vi "Unicode String Normalization Example.vi"() -> ()   [LabVIEW 2020]
doc: "This example demonstrates Unicode string normalization and compares the result of each of the normalization forms."
uses:
  Types/UTF-8 String/UTF-8 String.lvclass/UTF-8 String.ctl
  String/Controls/Normalized Form.ctl
  Dialog & User Interface/Polymorphic VIs/Write Control Text/Write String Value (UTF-8 String).vi
  Dialog & User Interface/Polymorphic VIs/Write Control Text/Write Ring Strings (UTF-8 String).vi
  87eab71b-edd1-4ab4-a82b-cc44d71eae5a.vi
  fbd87bf1-22c2-4bfe-9a71-b40242120771.vi
  c0d17205-3000-44ff-8427-9931fc65464d.vi
  1d2ce790-e22e-409d-a6eb-9d15f9dc24c3.vi
  2fb06fa7-1877-45b3-88e1-542f5745c524.vi
  90507d11-c02e-49ea-b453-6dce07ba0123.vi
  61f88bc1-4490-4656-bc91-370f28d961b2.vi
  2387616d-ad84-49dc-88c3-6113dd534e76.vi
  364c4283-3d14-4df8-9c3b-6263318f94ac.vi
  Unicode/Encode String.vi
  Dialog & User Interface/Polymorphic VIs/Write Control Text/Write String Value (UTF-8 String).vi/5206cb6b-04fb-41f5-a37e-29c14f142303.vi
  Private/Library/gu_codepoint_array_to_string.vi
  Types/UTF-8 String/Write Encoded UTF-8 String.vi
  Dialog & User Interface/Polymorphic VIs/Write Control Text/Write Ring Strings (UTF-8 String).vi/5206cb6b-04fb-41f5-a37e-29c14f142303.vi
  Private/Library/gu_normalize_string.vi
  Private/Conversion/String as Encoded String.vi
  Private/Conversion/Polymorphic VIs/String as Encoded String (UTF-8 String).vi
  Private/Library/gu_string_to_codepoint_array.vi
  Private/Conversion/Text to UTF-8.vi
  Private/Conversion/Polymorphic VIs/Text to UTF-8 (LabVIEW String).vi
  Private/Conversion/Encoded UTF-8 String to Encoded UTF-16LE String.vi
  Unicode/SubVIs/UTF-16 Byte Swap.vi
  Private/Conversion/UTF-8 to Text.vi
  Private/Conversion/Polymorphic VIs/UTF-8 to Text (LabVIEW String).vi
  Private/Conversion/Encoded UTF-16LE String to Encoded UTF-8 String.vi
  Unicode/Prepend BOM.vi
  Private/Conversion/Text as Encoded String.vi
  Private/Conversion/Polymorphic VIs/Text as Encoded String (UTF-8 String).vi
  Private/Library/Result To Error.vi
  Private/Memory/Copy String.vi
  Types/UTF-8 String/Read Encoded UTF-8 String.vi
  Private/Library/gu_string_to_codepoint_array.vi/5c793459-c97f-49eb-b871-f007f412847a.vi
  Unicode/SubVIs/Byte Order Marks.vi
  Unicode/Detect BOM.vi
  Private/Memory/Copy String.vi/4d47babd-4a2d-4eb7-b91b-7e707d692665.vi
  Private/Library/gu_free.vi
  Private/Library/gu_string_to_codepoint_array.vi/5c793459-c97f-49eb-b871-f007f412847a.vi/bf7dd0c3-7326-468c-a5c4-9eb034008d84.vi
  Unicode/Detect String Encoding.vi
  <vilib>/Utility/error.llb/Error Cluster From Error Code.vi
  Private/User Interface/Write Ring Control.vi
  Private/User Interface/Write String.vi
  Types/UTF-8 String/UTF-8 String.lvclass
  G-Unicode.lvlib
panel:
  out "Source":cluster{"Source":i32, "Source":string}[](array[cluster]) {"Source" format="%04x"}
  out "NFKD":cluster{"NFKD":i32, "NFKD":string}[](array[cluster]) {"NFKD" format="%04x"}
  out "NFKC":cluster{"NFKC":i32, "NFKC":string}[](array[cluster]) {"NFKC" format="%04x"}
  out "NFD":cluster{"NFD":i32, "NFD":string}[](array[cluster]) {"NFD" format="%04x"}
  out "NFC":cluster{"NFC":i32, "NFC":string}[](array[cluster]) {"NFC" format="%04x"}
  in  "Source":u16(ring) items=["+!", "&!", "Å", "ô", "i", "#", "q#", "û", "2u ", "›#"]
  out "NFKD":string
  out "NFKC":string
  out "NFD":string
  out "NFC":string
  # "Instructions:\n1. Run the VI, then select a Unicode string from the Source drop down.\n2. The string will be normalized into four different forms:\n    C - Composition\n    D - Decomposition\n    KC - Compatibility Composition\n    KD - Compatibility Decomposition\n3. Compare the string and codepoint values to see how the source string has been normalized.\n4. Detailed explanations of each normalization form and example can be found at https://unicode.org/reports/tr15/#Norm_Forms"
  # "G"
  # "-Unicode"
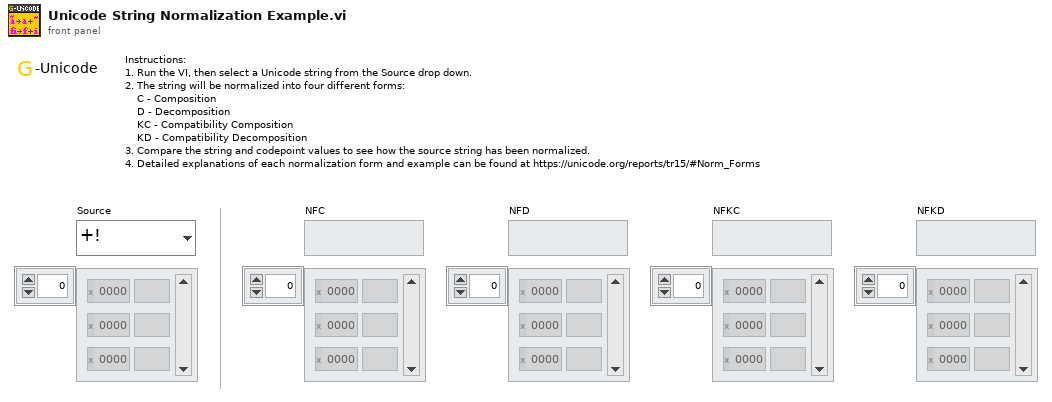
[diagram p1: front panel]
types:
  T1 = typedef "G-Unicode.lvlib/Normalized Form.ctl" = enum16{"C", "D", "KC", "KD"}
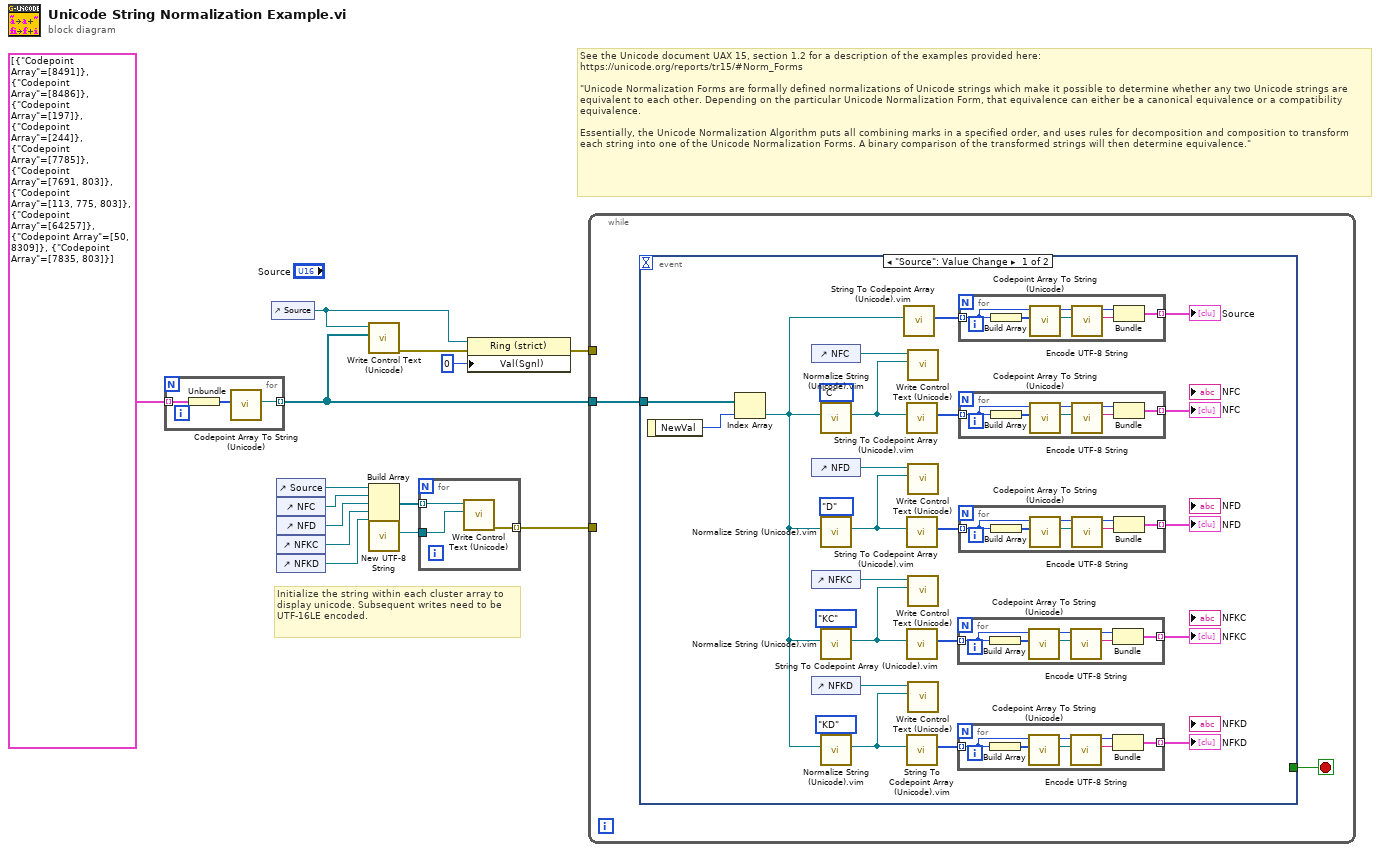
[diagram p0: block diagram]
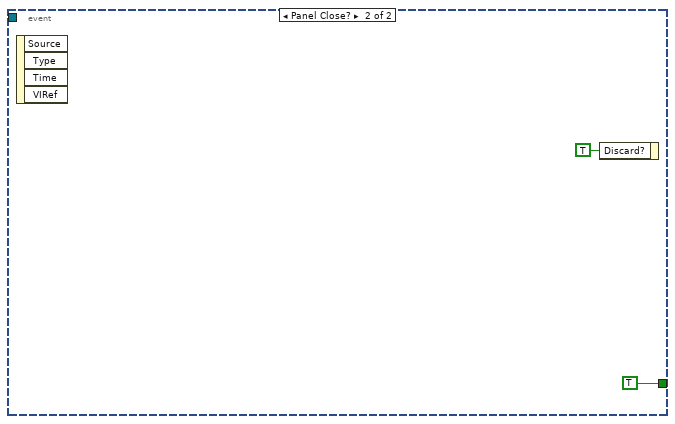
[diagram p2: hidden frame]
diagram:
  # "Initialize the string within each cluster array to display unicode. Subsequent writes need to be UTF-16LE encoded."
  # "See the Unicode document UAX 15, section 1.2 for a description of the examples provided here:\nhttps://unicode.org/reports/tr15/#Norm_Forms\n\n\"Unicode Normalization Forms are formally defined normalizations of Unicode strings which make it possible to determine whether any two Unicode strings are equivalent to each other. Depending on the particular Unicode Normalization Form, that equivalence can either be a canonical equivalence or a compatibility equivalence.\n\nEssentially, the Unicode Normalization Algorithm puts all combining marks in a specified order, and uses rules for decomposition and composition to transform each string into one of the Unicode Normalization Forms. A binary comparison of the transformed strings will then determine equivalence.\""
  n1 = for {
    tunnel: cluster{"Codepoint Array":i32[]}[] [{"Codepoint Array"=[8491]}, {"Codepoint Array"=[8486]}, {"Codepoint Array"=[197]}, {"Codepoint Array"=[244]}, {"Codepoint Array"=[7785]}, {"Codepoint Array"=[7691, 803]}, {"Codepoint Array"=[113, 775, 803]}, {"Codepoint Array"=[64257]}, {"Codepoint Array"=[50, 8309]}, {"Codepoint Array"=[7835, 803]}] -> [w17] mode=indexing
    tunnel: [w15] -> w9 mode=indexing
    n2 = Unbundle(w17) -> ("Codepoint Array"=w16:i32[])
    n3 = call "Codepoint Array To String (Unicode).vi"("Codepoint Array"=w16) -> ("String"=w15:refnum<class "UTF-8 String.lvclass">)  [unwired: 9 in, 1 out]
  }
  n4 = control-ref of="Source"() -> (w12:refnum<vi>)
  n5 = control-ref of="Source"() -> (w2:refnum<vi>)
  n6 = control-ref of="NFC"() -> (w8:refnum<vi>)
  n7 = control-ref of="NFD"() -> (w7:refnum<vi>)
  n8 = control-ref of="NFKC"() -> (w6:refnum<vi>)
  n9 = control-ref of="NFKD"() -> (w5:refnum<vi>)
  n10 = call-poly "Write Control Text (Unicode).vi"("Value"=w9, "Control Ref"=w12) -> ("error out"=w13:errorcluster)  [unwired: 9 in]
  n11 = Build Array(w2, w8, w7, w6, w5) -> (w4:refnum<vi>[])
  n12 = call "New UTF-8 String.vi"() -> ("UTF-8 String"=w3:refnum<class "UTF-8 String.lvclass">)  [unwired: 10 in, 1 out]
  n13 = for {
    tunnel: w4 -> [w20] mode=indexing
    tunnel: w3 -> [w19]
    tunnel: [w18] -> w1 mode=indexing
    n14 = call-poly "Write Control Text (Unicode).vi"("Value"=w19, "Control Ref"=w20) -> ("error out"=w18:errorcluster)  [unwired: 9 in]
  }
  n15 = property class="Ring (strict)"(reference=w12, error in=w13, "Val(Sgnl)"=u16 0 ("Value (Signaling)")) -> (error out=w10:errorcluster)  [unwired: 1 out]
  n16 = while {
    tunnel: w9 -> [w22]
    tunnel: w10 -> [_]
    tunnel: w1 -> [_]
    stop <- w21 stop-if-true
    n17 = event shown="[0] \"Source\": Value Change" {
      selector: _ -> [_ _]
      dyn-events: _ -> [_ _]
      timeout: _ -> [_ _]
      tunnel: w22 -> [w35 _]
      tunnel: [_ TRUE ("Discard?")] -> w21
      event "Source": Value Change {
        n18 = event-data() -> ("NewVal"=w34:u16)  [unwired: 1 in]
        n19 = Index Array(array=w35, index=w34) -> (element=w33:refnum<class "UTF-8 String.lvclass">)
        n20 = control-ref of="NFC"() -> (w45:refnum<vi>)
        n21 = control-ref of="NFD"() -> (w44:refnum<vi>)
        n22 = control-ref of="NFKC"() -> (w41:refnum<vi>)
        n23 = control-ref of="NFKD"() -> (w40:refnum<vi>)
        n24 = call "Normalize String (Unicode).vim"("Normalized Form (C)"=Normalized_Form."C", "String"=w33) -> ("Normalized String"=w39:refnum<class "UTF-8 String.lvclass">)  [unwired: 7 in, 1 out]
        n25 = call "Normalize String (Unicode).vim"("Normalized Form (C)"=Normalized_Form."D", "String"=w33) -> ("Normalized String"=w38:refnum<class "UTF-8 String.lvclass">)  [unwired: 7 in, 1 out]
        n26 = call "Normalize String (Unicode).vim"("Normalized Form (C)"=Normalized_Form."KC", "String"=w33) -> ("Normalized String"=w37:refnum<class "UTF-8 String.lvclass">)  [unwired: 7 in, 1 out]
        n27 = call "Normalize String (Unicode).vim"("Normalized Form (C)"=Normalized_Form."KD", "String"=w33) -> ("Normalized String"=w36:refnum<class "UTF-8 String.lvclass">)  [unwired: 7 in, 1 out]
        n28 = call "String To Codepoint Array (Unicode).vim"("String"=w33) -> ("Codepoint Array"=w27:i32[])  [unwired: 9 in, 1 out]
        n29 = call "String To Codepoint Array (Unicode).vim"("String"=w39) -> ("Codepoint Array"=w32:i32[])  [unwired: 9 in, 1 out]
        n30 = call "String To Codepoint Array (Unicode).vim"("String"=w38) -> ("Codepoint Array"=w30:i32[])  [unwired: 9 in, 1 out]
        n31 = call "String To Codepoint Array (Unicode).vim"("String"=w37) -> ("Codepoint Array"=w29:i32[])  [unwired: 9 in, 1 out]
        n32 = call "String To Codepoint Array (Unicode).vim"("String"=w36) -> ("Codepoint Array"=w28:i32[])  [unwired: 9 in, 1 out]
        n33 = call-poly "Write Control Text (Unicode).vi"("Value"=w39, "Control Ref"=w45) -> ()  [unwired: 9 in, 1 out]
        n34 = call-poly "Write Control Text (Unicode).vi"("Value"=w38, "Control Ref"=w44) -> ()  [unwired: 9 in, 1 out]
        n35 = call-poly "Write Control Text (Unicode).vi"("Value"=w37, "Control Ref"=w41) -> ()  [unwired: 9 in, 1 out]
        n36 = call-poly "Write Control Text (Unicode).vi"("Value"=w36, "Control Ref"=w40) -> ()  [unwired: 9 in, 1 out]
        n37 = for {
          tunnel: w29 -> [w59] mode=indexing
          tunnel: [w58] -> w24 mode=indexing
          n38 = Build Array(w59) -> (w62:i32[])
          n39 = call "Codepoint Array To String (Unicode).vi"("Codepoint Array"=w62) -> ("String"=w61:refnum<class "UTF-8 String.lvclass">)  [unwired: 9 in, 1 out]
          n40 = call "Encode UTF-8 String.vi"("UTF-8 String"=w61) -> ("Encoded String"=w60:string)  [unwired: 9 in, 1 out]
          n41 = Bundle("Type"=w59, "Encoded String"=w60) -> (w58:cluster{"Type":i32, "Encoded String":string})  [unwired: 1 in]
        }
        "NFKC" <- w24
        n42 = for {
          tunnel: w28 -> [w54] mode=indexing
          tunnel: [w53] -> w25 mode=indexing
          n43 = Build Array(w54) -> (w57:i32[])
          n44 = call "Codepoint Array To String (Unicode).vi"("Codepoint Array"=w57) -> ("String"=w56:refnum<class "UTF-8 String.lvclass">)  [unwired: 9 in, 1 out]
          n45 = call "Encode UTF-8 String.vi"("UTF-8 String"=w56) -> ("Encoded String"=w55:string)  [unwired: 9 in, 1 out]
          n46 = Bundle("Type"=w54, "Encoded String"=w55) -> (w53:cluster{"Type":i32, "Encoded String":string})  [unwired: 1 in]
        }
        "NFKD" <- w25
        n47 = for {
          tunnel: w27 -> [w49] mode=indexing
          tunnel: [w48] -> w23 mode=indexing
          n48 = Build Array(w49) -> (w52:i32[])
          n49 = call "Codepoint Array To String (Unicode).vi"("Codepoint Array"=w52) -> ("String"=w51:refnum<class "UTF-8 String.lvclass">)  [unwired: 9 in, 1 out]
          n50 = call "Encode UTF-8 String.vi"("UTF-8 String"=w51) -> ("Encoded String"=w50:string)  [unwired: 9 in, 1 out]
          n51 = Bundle("Type"=w49, "Encoded String"=w50) -> (w48:cluster{"Type":i32, "Encoded String":string})  [unwired: 1 in]
        }
        "Source" <- w23
        n52 = for {
          tunnel: w32 -> [w69] mode=indexing
          tunnel: [w68] -> w31 mode=indexing
          n53 = Build Array(w69) -> (w72:i32[])
          n54 = call "Codepoint Array To String (Unicode).vi"("Codepoint Array"=w72) -> ("String"=w71:refnum<class "UTF-8 String.lvclass">)  [unwired: 9 in, 1 out]
          n55 = call "Encode UTF-8 String.vi"("UTF-8 String"=w71) -> ("Encoded String"=w70:string)  [unwired: 9 in, 1 out]
          n56 = Bundle("Type"=w69, "Encoded String"=w70) -> (w68:cluster{"Type":i32, "Encoded String":string})  [unwired: 1 in]
        }
        "NFC" <- w31
        n57 = for {
          tunnel: w30 -> [w64] mode=indexing
          tunnel: [w63] -> w26 mode=indexing
          n58 = Build Array(w64) -> (w67:i32[])
          n59 = call "Codepoint Array To String (Unicode).vi"("Codepoint Array"=w67) -> ("String"=w66:refnum<class "UTF-8 String.lvclass">)  [unwired: 9 in, 1 out]
          n60 = call "Encode UTF-8 String.vi"("UTF-8 String"=w66) -> ("Encoded String"=w65:string)  [unwired: 9 in, 1 out]
          n61 = Bundle("Type"=w64, "Encoded String"=w65) -> (w63:cluster{"Type":i32, "Encoded String":string})  [unwired: 1 in]
        }
        "NFD" <- w26
      }
      event Panel Close? {
        n62 = event-data() -> ()  [unwired: 1 in, 4 out]
        n63 = event-data("Discard?"=TRUE) -> ()  [unwired: 1 in, 1 out]
      }
    }
  }
